vi "Capacitance_IS_CalculateZDut.vi"(7 "Data Id":string, 9 "ZRef Im":dbl[](array[numeric]), 10 "ZRef Real":dbl[](array[numeric]), 11 "Semiconductor Module Context":T1) -> (0 "error out":errorcluster)   [LabVIEW 2023, in "Capacitance.lvlib"]
doc: "Calculates ZDut=Zref*(V1-V2)/V2"
uses:
  Capacitance.lvlib
  <vilib>/NI_TestStand_SemiconductorModule/NI_TestStand_Semiconductor_Module.lvlibp/PinMap/General/SemiconductorModuleContext.ctl
  <vilib>/NI_TestStand_SemiconductorModule/NI_TestStand_Semiconductor_Module.lvlibp
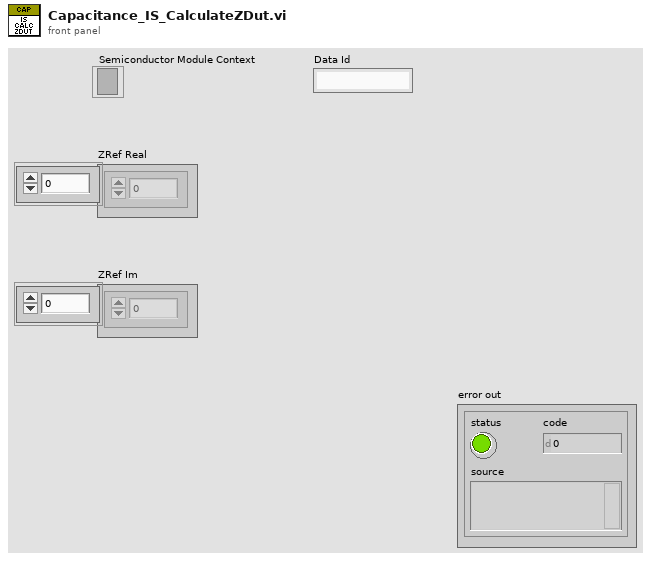
[diagram p1: front panel]
types:
  T1 = typedef "NI_TestStand_Semiconductor_Module.lvlibp/SemiconductorModuleContext.ctl" = refnum<k7>
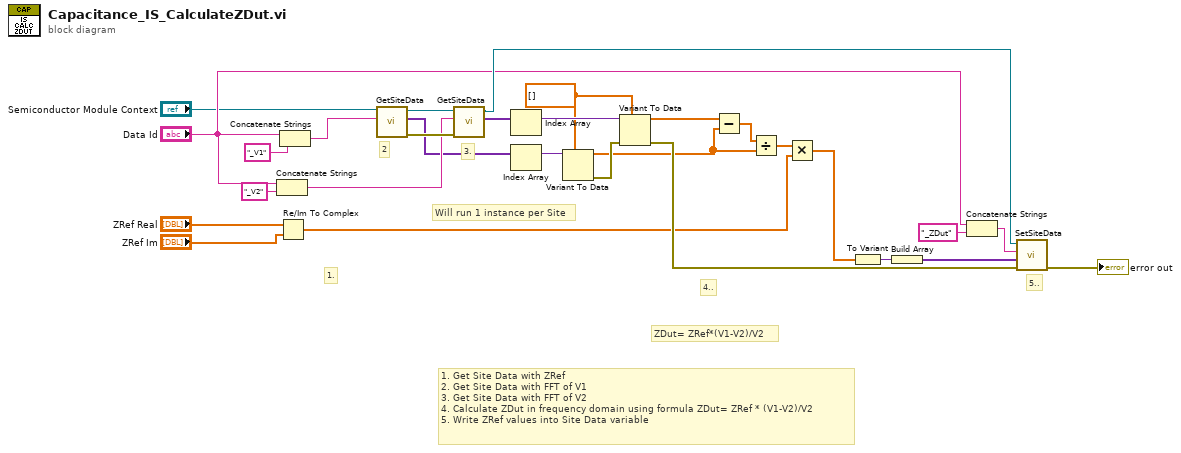
[diagram p0: block diagram]
diagram:
  w11 = cdb[] []
  # "Will run 1 instance per Site"
  # "4.."
  # "3."
  # "1. Get Site Data with ZRef\n2. Get Site Data with FFT of V1\n3. Get Site Data with FFT of V2\n4. Calculate ZDut in frequency domain using formula ZDut= ZRef * (V1-V2)/V2\n5. Write ZRef values into Site Data variable"
  # "5.."
  # "2"
  # "1."
  # "ZDut= ZRef*(V1-V2)/V2"
  n1 = Concatenate Strings("Data Id", "_V2" ("string")) -> (w24:string)
  n2 = Re/Im To Complex(1:"ZRef Im", 2:"ZRef Real") -> (0:w3:cdb[])
  n3 = Concatenate Strings("Data Id", "_V1" ("string")) -> (w29:string)
  n4 = call <vilib>:"GetSiteData.vi"("Data Id"=w29, "Semiconductor Module Context"="Semiconductor Module Context") -> ("error out"=w27:errorcluster, "Site Data"=w22:variant[], "Semiconductor Module Context Out"=w28:T1)  [unwired: 7 in]
  n5 = call <vilib>:"GetSiteData.vi"("error in (no error)"=w27, "Data Id"=w24, "Semiconductor Module Context"=w28) -> ("Site Data"=w23:variant[], "Semiconductor Module Context Out"=w20:T1)  [unwired: 6 in, 1 out]
  n6 = Index Array(array=w23) -> (element=w15:variant)  [unwired: 1 in]
  n7 = Index Array(array=w22) -> (element=w14:variant)  [unwired: 1 in]
  n8 = Variant To Data(type=w11, Variant=w14) -> (data=w9:cdb[], error out=w13:errorcluster)  [unwired: 1 in]
  n9 = Variant To Data(error in=w13, type=w11, Variant=w15) -> (data=w12:cdb[], error out=w21:errorcluster)
  n10 = Subtract(x=w12, y=w9) -> (x-y=w10:cdb[])
  n11 = Divide(x=w10, y=w9) -> (x/y=w8:cdb[])
  n12 = Multiply(x=w8, y=w3) -> (x*y=w7:cdb[])
  n13 = To Variant(anything=w7) -> (Variant=w2:variant)
  n14 = Build Array(w2) -> (w1:variant[])
  n15 = Concatenate Strings("Data Id", "_ZDut" ("string")) -> (w19:string)
  n16 = call <vilib>:"SetSiteData.vi"("error in (no error)"=w21, "Site Data"=w1, "Data Id"=w19, "Semiconductor Module Context"=w20) -> ("error out"=→"error out":errorcluster)  [unwired: 5 in, 1 out]
